vi "{{Msg}}.vi"(6 "Error":errorcluster, 7 "ActorMsg":refnum<class "ActorMsg.lvclass">, 11 "Msg":refnum<class "Msg.lvclass">) -> (3 "Msg":refnum<class "Msg.lvclass">, 4 "Error":errorcluster, 5 "ActorMsg":refnum<class "ActorMsg.lvclass">)   [LabVIEW 2020, in "_Template.lvlib" / "{{Msg}}.lvlib" / "ActorMsg.lvclass"]
uses:
  ActorMsg.lvclass
  Msg/Msg.lvclass
panel:
  # "This front panel should not be manipulated."
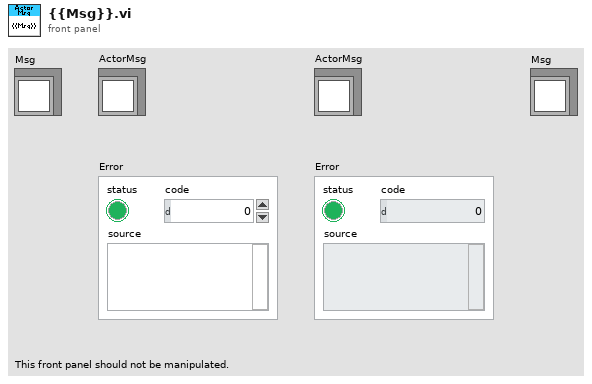
[diagram p1: front panel]
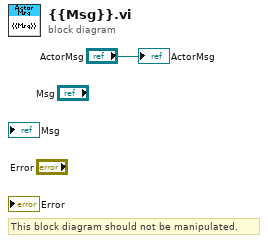
[diagram p0: block diagram]
diagram:
  # "This block diagram should not be manipulated."
  "ActorMsg" <- "ActorMsg"
